vi "test Verify CLI STD ERR .vi"(8 "error in":errorcluster, 11 "Test Case In":refnum<class "LUnit Extensions Tests.lvclass">) -> (0 "error out":errorcluster, 3 "Test Case Out":refnum<class "LUnit Extensions Tests.lvclass">)   [LabVIEW 2020, in "LUnit Extensions Tests.lvclass"]
uses:
  LUnit Extensions Tests.lvclass
  LUnit Extensions Tests.lvclass/LUnit Extensions Tests.ctl
  C:/Program Files/National Instruments/LabVIEW 2026/vi.lib/Astemes/LUnit/Test Case.lvclass
  C:/Program Files/National Instruments/LabVIEW 2026/vi.lib/Astemes/LUnit/LUnit Runnable.lvclass
  C:/Users/SAS/Desktop/ApprovalTests.LabVIEW/Tests/LUnit.Tests/LUnit Extensions Tests/LUnit Extensions Tests.lvclass
  Source/Extensions/LUnit.Extension/LUnit.Extension.lvlib
  Source/Approval Tests/Approval Tests.lvlib
  Source/Approval Tests/OS Strings.ctl
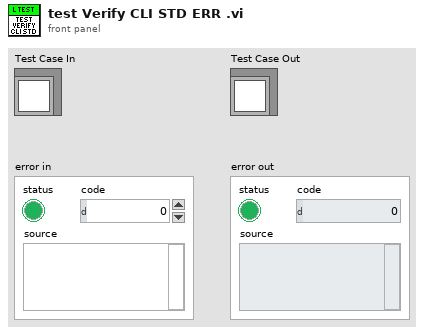
[diagram p1: front panel]
types:
  T1 = typedef "Approval Tests.lvlib/OS Strings.ctl" = cluster{"Windows":string, "Linux":string, "Mac":string}
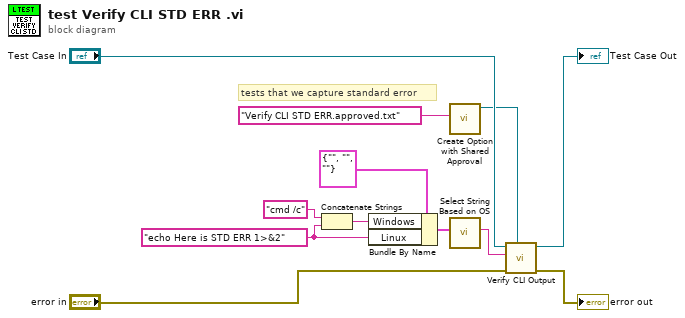
[diagram p0: block diagram]
diagram:
  w1 = "echo Here is STD ERR 1>&2" ("command line")
  # "tests that we capture standard error"
  n1 = Concatenate Strings("cmd /c" ("string"), w1) -> (w2:string)
  n2 = Bundle By Name(cluster=T1 {"Windows"="", "Linux"="", "Mac"=""} ("Strings"), "Windows"=w2, "Linux"=w1) -> (w3:T1)
  n3 = call "Create Option with Shared Approval.vi"("Filename"="Verify CLI STD ERR.approved.txt") -> ("Options outs"=w8:refnum<class "Options.lvclass">)  [unwired: 10 in]
  n4 = call "Select String Based on OS.vi"("Strings"=w3) -> ("Selection"=w5:string)  [unwired: 10 in]
  n5 = call "Verify CLI Output.vi"("Options"=w8, "error in"="error in", "command line"=w5, "LUnit Test Case In"="Test Case In") -> ("error out"=→"error out":errorcluster, "LUnit Test Case Out"=→"Test Case Out":refnum<class "LUnit Extensions Tests.lvclass">)  [unwired: 6 in]
